vi "Yscaling_flt.vi"(6 "Scaling?":bool, 10 "Y":dbl, 11 "Plane Height":dbl) -> (3 "y scaled":dbl, 4 "output cluster":T1)   [LabVIEW 2019]
uses:
  GlobalClicksHeight_flt.vi
  <userlib>/HapticSTM/HapticSTM.lvlib
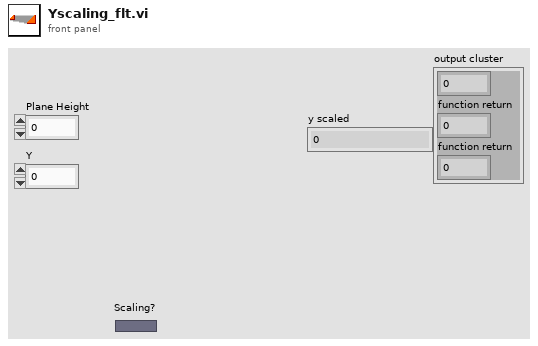
[diagram p1: front panel]
types:
  T1 = cluster{dbl, "function return":dbl, "function return":dbl}
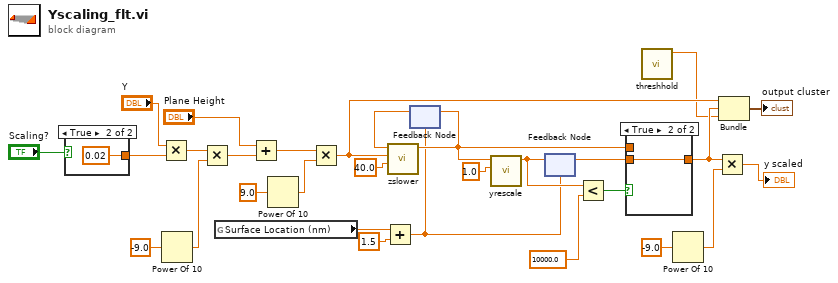
[diagram p0: block diagram]
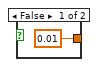
[diagram p2: hidden frame]
diagram:
  n1 = case shown="True" "Scaling?" {
    tunnel: [0.01 ("y") 0.02 ("y")] -> w3
    frame False {
    }
    frame True {
    }
  }
  n2 = Multiply(x="Y", y=w3) -> (x*y=w25:dbl)
  n3 = Power Of 10(x=-9.0) -> (10^x=w24:dbl)
  n4 = Multiply(x=w25, y=w24) -> (x*y=w26:dbl)
  n5 = global read "GlobalClicksHeight_flt.vi" "Surface Location (nm)"() -> (w8:dbl)
  n6 = Add(x="Plane Height", y=w26) -> (x+y=w29:dbl)
  n7 = Power Of 10(x=9.0) -> (10^x=w28:dbl)
  n8 = Multiply(x=w29, y=w28) -> (x*y=w11:dbl)
  n9 = Add(x=w8, y=1.5) -> (x+y=w6:dbl)
  n10 = feedback #1(w6) -> (w12:dbl)
  n11 = call <userlib>:"zslower.vi"("maxvel"=40.0, "labview_zpos_write"=w11, "nanonis_zpos_read"=w12) -> ("function return"=w9:dbl)  [unwired: 8 in]
  n12 = feedback-in #1(w9) -> ()
  n13 = call <userlib>:"yrescale.vi"("scalingfactor"=1.0, "ylabview"=w9) -> ("function return"=w10:dbl)  [unwired: 9 in]
  n14 = feedback-in #2(w10) -> ()
  n15 = feedback #2(w6) -> (w14:dbl)
  n16 = Less?(x=w10, y=10000.0) -> (x < y?=w15:bool)
  n17 = case shown="True" w15 {
    tunnel: [w32 w33] -> w5
    tunnel: w14 -> [_ w33]
    tunnel: w9 -> [w32 _]
    frame False {
    }
    frame True {
    }
  }
  n18 = call <userlib>:"threshhold.vi"() -> ("function return"=w2:dbl)  [unwired: 11 in]
  n19 = Power Of 10(x=-9.0) -> (10^x=w19:dbl)
  n20 = Multiply(x=w5, y=w19) -> (x*y=→"y scaled":dbl)
  n21 = Bundle(w11, "function return"=w5, "function return"=w2) -> (→"output cluster":T1)  [unwired: 1 in]
